vi "Take N.vi"(10 "N":i32, 11 "arr":dbl[](array[numeric])) -> (3 "stuff out":dbl[](array[numeric]))   [LabVIEW 2019]
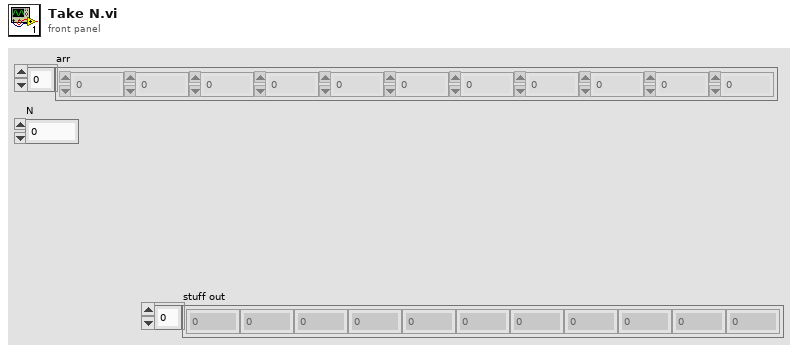
[diagram p1: front panel]
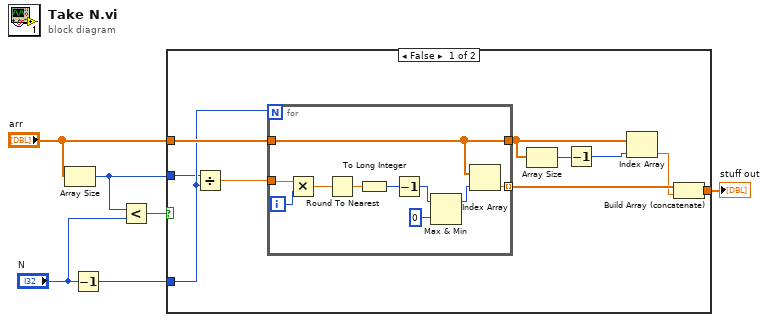
[diagram p0: block diagram]
diagram:
  n1 = Array Size(array="arr") -> (size(s)=w3:i32)
  n2 = Decrement(x="N") -> (x-1=w5:i32)
  n3 = Less?(x=w3, y="N") -> (x < y?=w1:bool)
  n4 = case shown="False" w1 {
    tunnel: "arr" -> [w15 w27]
    tunnel: w5 -> [w14 _]
    tunnel: [w8 w27] -> w4
    tunnel: w3 -> [w7 _]
    frame False {
      n5 = Divide(x=w7, y=w14) -> (x/y=w16:dbl)
      n6 = for {
        N: w14 -> [_]
        tunnel: w16 -> [w26]
        tunnel: w15 -> [w17]
        tunnel: [w22] -> w13 mode=indexing
        tunnel: [w17] -> w12
        i -> [w25]
        n7 = Multiply(x=w26, y=w25) -> (x*y=w24:dbl)
        n8 = Round To Nearest(number=w24) -> (nearest integer value=w23:dbl)
        n9 = To Long Integer(number=w23) -> (32bit integer=w21:i32)
        n10 = Decrement(x=w21) -> (x-1=w20:i32)
        n11 = Max & Min(x=w20, y=0) -> (max(x,y)=w18:i32)  [unwired: 1 out]
        n12 = Index Array(array=w17, index=w18) -> (element=w22:dbl)
      }
      n13 = Array Size(array=w12) -> (size(s)=w11:i32)
      n14 = Decrement(x=w11) -> (x-1=w10:i32)
      n15 = Index Array(array=w12, index=w10) -> (element=w9:dbl)
      n16 = Build Array (concatenate)(w13, w9) -> (w8:dbl[])
    }
    frame True {
    }
  }
  "stuff out" <- w4
